vi "get-child-tags-by-id.vi"(8 "error in (no error)":errorcluster, 10 "id":u32, 11 "CANtable in":refnum<class "bAPPdata.lvclass">) -> (0 "error out":errorcluster, 2 "child.rags":string[](array[string]), 3 "CANtable out":refnum<class "bAPPdata.lvclass">)   [LabVIEW 2015, in "bAPPdata.lvclass"]
uses:
  class.can.table/bAPPdata.lvclass
  class.can.table/bAPPdata.lvclass/bAPPdata.ctl
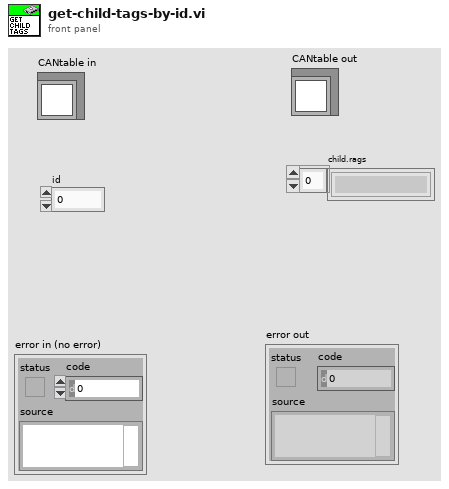
[diagram p1: front panel]
types:
  T1 = typedef "bAPPdata.lvclass/table-data.ctl" = T2[]
  T2 = typedef "bAPPdata.lvclass/table-contents.ctl" = cluster{"id":u32, "tag":string, "frame.type":T3, "last.frame":T4, "tMsgData":T6, "child.tags":string[], "bit-payload":bool[]}
  T3 = typedef "frame.type.ctl" = enum16{"FRAME NOT DEFINED", "DUT OUTPUT FRAME", "DUT INPUT FRAME"}
  T4 = typedef "XNET Frame CAN.ctl" = cluster{"timestamp":timestamp, "payload":u8[], "identifier":u32, "type":T5, "extended?":bool, "echo?":bool}
  T5 = typedef "XNET Frame Type CAN.ctl" = u8
  T6 = typedef "nMsgData.ctl" = cluster{"dwID":u32, "count":u32, "dwCycleTime":dbl, "dwTime":dbl, "new msg":bool}
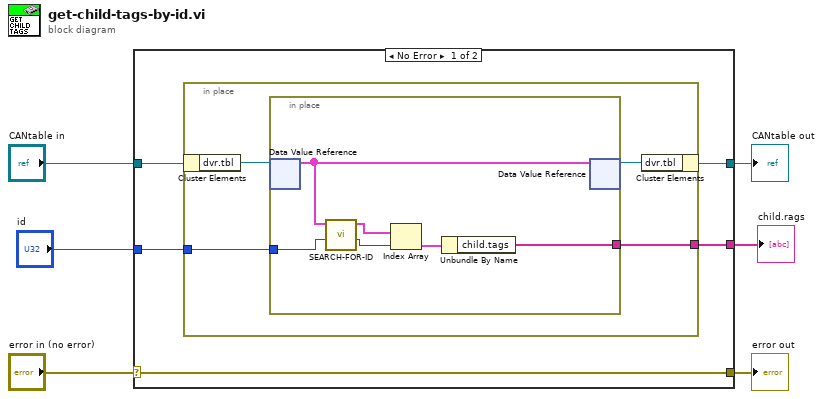
[diagram p0: block diagram]
diagram:
  n1 = case shown="No Error" "error in (no error)" {
    selector: "error in (no error)" -> [w11 w23]
    tunnel: [w11 w23] -> w5
    tunnel: [w9 w22] -> w3
    tunnel: "CANtable in" -> [w10 w22]
    tunnel: "id" -> [w8 _]
    tunnel: [w7 _] -> w1
    frame No Error {
      n2 = in-place {
        in-place-border: w8 -> [w13]
        in-place-border: [w12] -> w7
        n3 = in-place-cluster #1(w10) -> ("dvr.tbl"=w15:refnum<data-value>)
        n4 = in-place {
          in-place-border: w13 -> [w21]
          in-place-border: [w16] -> w12
          n5 = in-place-dvr #2(w15) -> (w20:T1)  [unwired: 1 out]
          n6 = call "SEARCH-FOR-ID.vi"("ID"=w21, "tbl.list"=w20) -> ("idx"=w19:i32, "tbl.list out"=w18:T2[])  [unwired: 8 in]
          n7 = Index Array(array=w18, index=w19) -> (element=w17:T2)
          n8 = Unbundle By Name(w17) -> ("child.tags"=w16:string[])
          n9 = in-place-dvr #2(w20) -> (w14:refnum<data-value>)  [unwired: 1 out]
        }
        n10 = in-place-cluster #1("dvr.tbl"=w14) -> (w9:refnum<class "bAPPdata.lvclass">)
      }
    }
    frame Error {
    }
  }
  "error out" <- w5
  "CANtable out" <- w3
  "child.rags" <- w1
